vi "SS Instrument Object Panel Ref.vi"(8 "error in (no error)":errorcluster, 10 "Config File Path":path, 11 "system settings":T1) -> (0 "error out":errorcluster)   [LabVIEW 2019]
uses:
  SS typedef cluster Instrument Cmd Q Init Parameters.ctl
panel:
  # "This VI created only to give a template for the connector pane for\ninstrument objects. Do not modify."
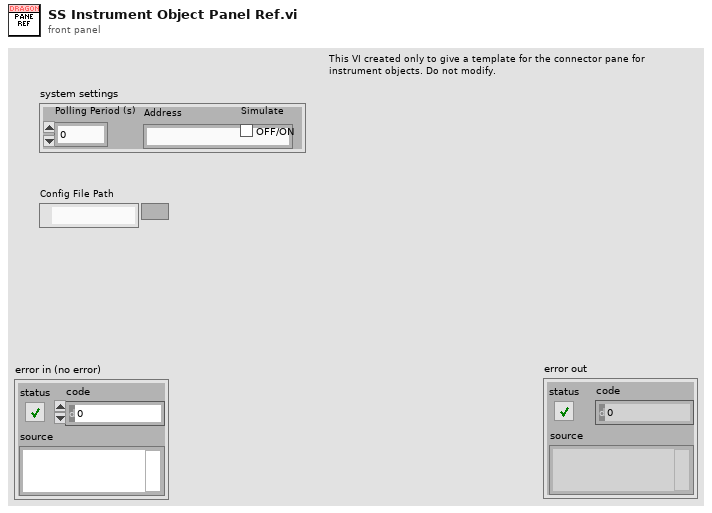
[diagram p1: front panel]
types:
  T1 = typedef "SS typedef cluster Instrument Cmd Q Init Parameters.ctl" = cluster{"Polling Period (s)":dbl, "Address":string, "Simulate":bool}
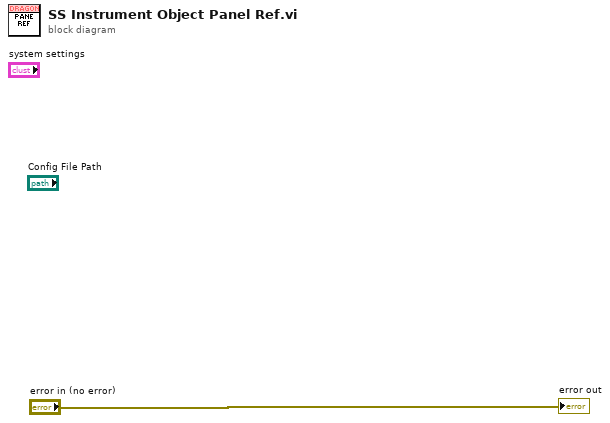
[diagram p0: block diagram]
diagram:
  "error out" <- "error in (no error)"
